vi "Connect to Server.vi"(8 "error in (no error)":errorcluster, 11 "url":string) -> (0 "error out":errorcluster, 3 ".NET Refnum out":refnum<k24>)   [LabVIEW 2024, in "LV_OPC_NET.lvlib"]
uses:
  C:/Users/Andrey/Desktop/LV_OPC-Client-x64/LV_OPC_Test/OPC.NET/OpcNetApi.dll
  OpcNetApi.dll
  C:/Users/Andrey/Desktop/LV_OPC-Client-x64/LV_OPC_Test/OPC.NET/OpcNetApi.Com.dll
  OpcNetApi.Com.dll
  LV_OPC_NET.lvlib
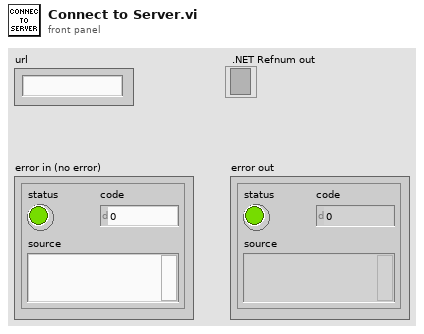
[diagram p1: front panel]
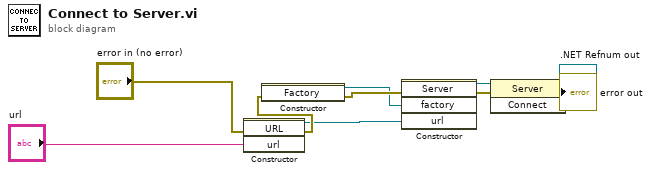
[diagram p0: block diagram]
diagram:
  n1 = constructor class="URL"(error in="error in (no error)", "url"="url") -> (reference out=w1:refnum<k24>, error out=w7:errorcluster)  [unwired: 2 in, 2 out]
  n2 = constructor class="Factory"(error in=w7) -> (reference out=w5:refnum<k24>, error out=w8:errorcluster)  [unwired: 2 in, 1 out]
  n3 = constructor class="Server"(error in=w8, "factory"=w5, "url"=w1) -> (reference out=w2:refnum<k24>, error out=w9:errorcluster)  [unwired: 2 in, 3 out]
  n4 = invoke class="Server" method="Connect"(reference=w2, error in=w9) -> (reference out=→".NET Refnum out":refnum<k24>, error out=→"error out":errorcluster)  [unwired: 1 in, 1 out]
